vi "StringToNumber.vi"(1 "String":string) -> (0 "Output":dbl)   [LabVIEW 2019]
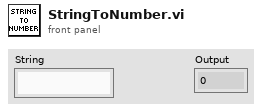
[diagram p1: front panel]
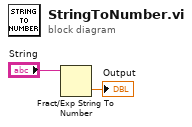
[diagram p0: block diagram]
diagram:
  n1 = Fract/Exp String To Number(string="String") -> (number=→"Output":dbl)  [unwired: 3 in, 1 out]
